vi "Get Config File Path.vi"(8 "error in (no error)":errorcluster) -> (0 "error out":errorcluster, 3 "Config Directory":path)   [LabVIEW 2020, in "Utilities.lvlib"]
doc: "Generates the default configuration path. \nWhen called from the development environement, the default config path is the /Config relative to the project path.\nWhen called from a built exe the default config path is at C:\\Users\\<username>\\AppData\\Local\\<CompanyName>\\<ProductName> where company name and product name are the ones configured in the build specification.\nOn Linux the default config directory is \\home\\lvuser\\natinst\\bin\\config."
uses:
  Utilities.lvlib
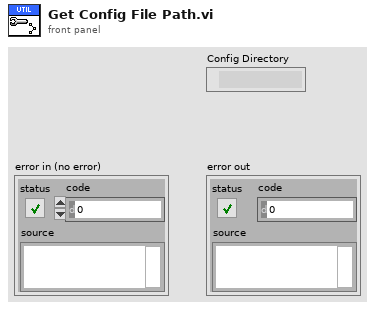
[diagram p1: front panel]
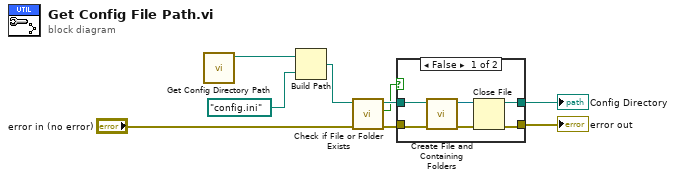
[diagram p0: block diagram]
diagram:
  n1 = call "Get Config Directory Path.vi"() -> ("appended path"=w3:path)  [unwired: 11 in]
  n2 = Build Path(base path=w3, name or relative path=path "config.ini") -> (appended path=w2:path)
  n3 = call <vilib>:"Check if File or Folder Exists.vi"("error in (no error)"="error in (no error)", "path"=w2) -> ("error out"=w5:errorcluster, "file or folder exists?"=w4:bool, "dup path"=w6:path)  [unwired: 7 in]
  n4 = case shown="False" w4 {
    tunnel: [w13 w16] -> w9
    tunnel: [w12 w17] -> w7
    tunnel: w6 -> [w11 w17]
    tunnel: w5 -> [w10 w16]
    frame False {
      n5 = call <vilib>:"Create File and Containing Folders.vi"("error in (no error)"=w10, "file path"=w11) -> ("error out"=w14:errorcluster, "refnum out"=w15:refnum<file>)  [unwired: 8 in]
      n6 = Close File(refnum=w15, error in=w14) -> (path=w12:path, error out=w13:errorcluster)
    }
    frame True {
    }
  }
  "Config Directory" <- w7
  "error out" <- w9
